vi "Generate and Launch HTML.vi"(8 "error in":errorcluster, 11 "Path":path=path "Auto - for reportting") -> (0 "error out":errorcluster)   [LabVIEW 2013]
uses:
  <vilib>/Platform/browser.llb/Open URL in Default Browser (path).vi
  <vilib>/regexp/Match Regular Expression.xnode
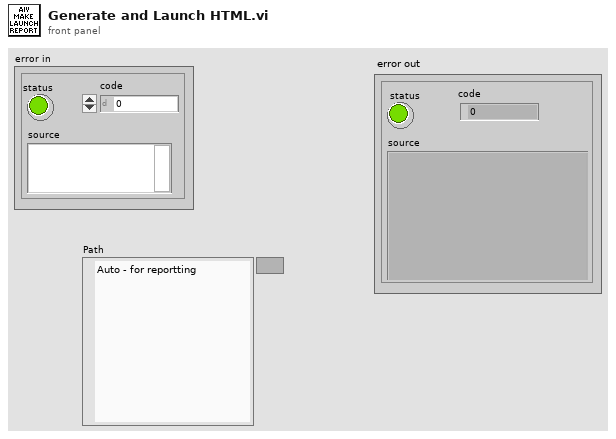
[diagram p1: front panel]
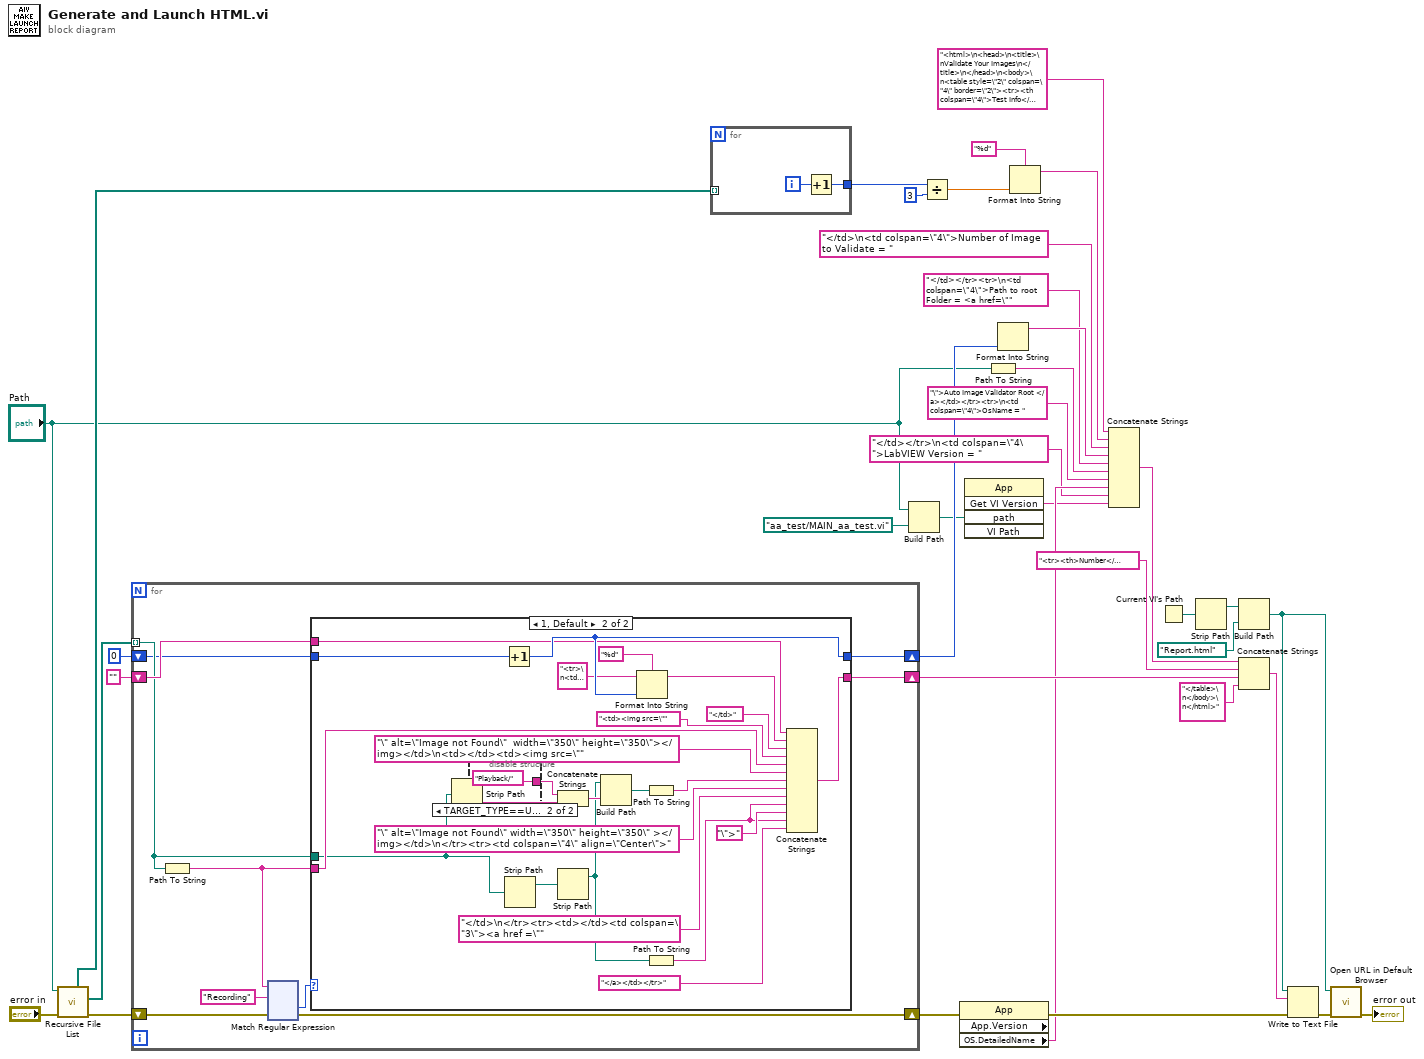
[diagram p0: block diagram]
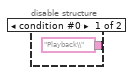
[diagram p3: hidden frame]
diagram:
  n1 = call <vilib>:"Recursive File List.vi"("error in (no error)"="error in", "Folder Path"="Path") -> ("error out"=w25:errorcluster, "All Files in Dir"=w37:path[], "All Folders"=w24:path[])  [unwired: 5 in, 2 out]
  n2 = for {
    tunnel: w37 -> [w40] mode=indexing
    shift-right: [w44] -> w36
    shift-left: "" -> [w43]
    shift-right: [w41] -> w20
    shift-left: w25 -> [w42]
    shift-right: [w39] -> w22
    shift-left: 0 -> [w38]
    n3 = Path To String(path=w40) -> (string=w45:string)
    n4 = xnode "Match Regular Expression"("input string"=w45, "regular expression"="Recording", "error in"=w42) -> ("offset past match"=w46:i32, "error out"=w41:errorcluster)  [unwired: 3 in, 3 out]
    n5 = case shown="1, Default" w46 {
      tunnel: w45 -> [_ w72]
      tunnel: [w49 w71] -> w44
      tunnel: w43 -> [w49 w57]
      tunnel: w40 -> [_ w54]
      tunnel: w38 -> [w48 w61]
      tunnel: [w48 w60] -> w39
      frame -1 {
      }
      frame 1, Default {
        n6 = Strip Path(path=w54) -> (name=w64:string)  [unwired: 1 out]
        n7 = disable-structure shown="TARGET_TYPE==Unix" {
          disable-tunnel: ["Playback\\" ("string") "Playback/" ("string")] -> w63
          frame condition #0 {
          }
          frame condition #1 (active) {
          }
        }
        n8 = Increment(x=w61) -> (x+1=w60:i32)
        n9 = Strip Path(path=w54) -> (stripped path=w69:path)  [unwired: 1 out]
        n10 = Concatenate Strings(w63, w64) -> (w62:string)
        n11 = Strip Path(path=w69) -> (stripped path=w50:path)  [unwired: 1 out]
        n12 = Build Path(base path=w50, name or relative path=w62) -> (appended path=w68:path)
        n13 = Format Into String(format string="%d", initial string="<tr>\n<td>", w60) -> (resulting string=w56:string)  [unwired: 1 in, 1 out]
        n14 = Path To String(path=w68) -> (string=w67:string)
        n15 = Path To String(path=w50) -> (string=w52:string)
        n16 = Concatenate Strings(w57, w56, "</td>" ("string"), "<td><img src=\"", w72, "\" alt=\"Image not Found\"  width=\"350\" height=\"350\"></img></td>\n<td></td><td><img src=\"" ("string"), w67, "\" alt=\"Image not Found\" width=\"350\" height=\"350\" ></img></td>\n</tr><tr><td colspan=\"4\" align=\"Center\">" ("string"), "</td>\n</tr><tr><td></td><td colspan=\"3\"><a href =\"" ("string"), w52, "\">" ("string"), w52, "</a></td></tr>" ("string")) -> (w71:string)
      }
    }
  }
  n17 = for {
    tunnel: w24 -> [_] mode=indexing
    tunnel: [w187] -> w23
    i -> [w188]
    n18 = Increment(x=w188) -> (x+1=w187:i32)
  }
  n19 = Build Path(base path="Path", name or relative path=path "aa_test/MAIN_aa_test.vi" ("appended path")) -> (appended path=w3:path)
  n20 = Divide(x=w23, y=3) -> (x/y=w9:dbl)
  n21 = property class="App" props=["App.Version", "OS.DetailedName"](error in=w20) -> (error out=w19:errorcluster, "OS.DetailedName"=w12:string)  [unwired: 1 in, 2 out]
  n22 = invoke class="App" method="Get VI Version"("path"=w3) -> ("GetVIVers"=w2:string)  [unwired: 4 in, 4 out]
  n23 = Path To String(path="Path") -> (string=w14:string)
  n24 = Format Into String(w22) -> (resulting string=w16:string)  [unwired: 3 in, 1 out]
  n25 = Format Into String(format string="%d", w9) -> (resulting string=w18:string)  [unwired: 2 in, 1 out]
  n26 = Concatenate Strings("<html>\n<head>\n<title>\nValidate Your Images\n</title>\n</head>\n<body>\n<table style=\"2\" colspan=\"4\" border=\"2\"><tr><th colspan=\"4\">Test Info</th></tr>\n<tr><td colspan=\"2\"> Number of Test Folder = " ("string"), w18, "</td>\n<td colspan=\"4\">Number of Image to Validate = ", w16, "</td></tr><tr>\n<td colspan=\"4\">Path to root Folder = <a href=\"" ("string"), w14, "\">Auto Image Validator Root </a></td></tr><tr>\n<td colspan=\"4\">OsName = " ("string"), w12, "</td></tr>\n<td colspan=\"4\">LabVIEW Version = " ("string"), w2) -> (w10:string)
  n27 = Current VI's Path() -> (path=w31:path)
  n28 = Strip Path(path=w31) -> (stripped path=w32:path)  [unwired: 1 out]
  n29 = Build Path(base path=w32, name or relative path=path "Report.html") -> (appended path=w30:path)
  n30 = Concatenate Strings(w10, "<tr><th>Number</th><th>RecordingImage</th><th></th><th>Playback Image</th></tr>" ("string"), w36, "</table>\n</body>\n</html>" ("string")) -> (w34:string)
  n31 = Write to Text File(file (use dialog)=w30, text=w34, error in=w19) -> (error out=w29:errorcluster)  [unwired: 1 in, 2 out]
  n32 = call-poly <vilib>:"Open URL in Default Browser.vi"("error in (no error)"=w29, "URL"=w30) -> ("error out"=→"error out":errorcluster)  [unwired: 4 in, 1 out]
